vi "ReplaceAllRows_lastrow.vi"(2 "Array in":dbl[][](array[numeric])=[[0.0, 1.0, 2.0], [0.0, 0.0, 0.0], [0.0, 0.0, 0.0], [5.0, 6.0, 7.0]]) -> (0 "Array out":dbl[][](array[numeric])=[[5.0, 6.0, 7.0], [5.0, 6.0, 7.0], [5.0, 6.0, 7.0], [5.0, 6.0, 7.0]])   [LabVIEW 2018]
panel:
  out "last row":dbl[][](array[numeric])=[[5.0, 6.0, 7.0]]
  out "other rows":dbl[][](array[numeric])=[[0.0, 1.0, 2.0], [0.0, 0.0, 0.0], [0.0, 0.0, 0.0]]
  # "the point of this VI is\nto make all rows the same as the last row\nso that anything not modified later is not changed during the ramp"
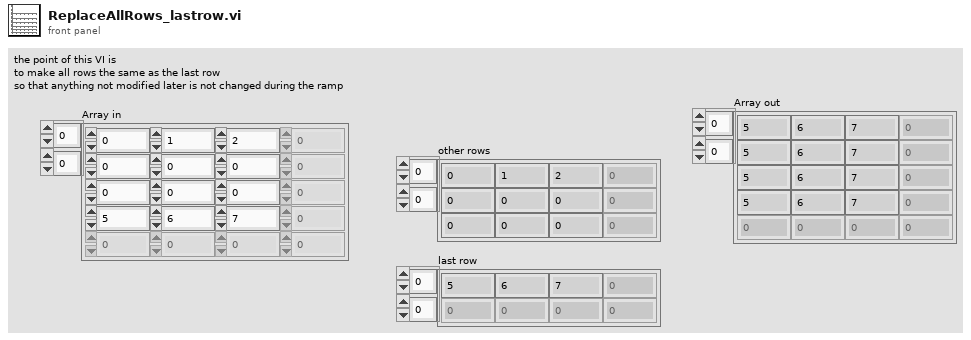
[diagram p1: front panel]
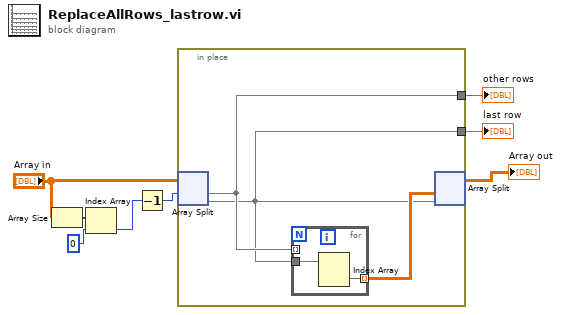
[diagram p0: block diagram]
diagram:
  n1 = Array Size(array="Array in") -> (size(s)=w3:i32[])
  n2 = Index Array(array=w3, index=0) -> (element=w1:i32)
  n3 = Decrement(x=w1) -> (x-1=w5:i32)
  n4 = in-place {
    in-place-border: [w10] -> w7
    in-place-border: [w9] -> w6
    n5 = in-place-split #1("Array in", w5) -> (w10:dbl[][], w9:dbl[][])
    n6 = for {
      tunnel: w10 -> [_] mode=indexing
      tunnel: w9 -> [w13]
      tunnel: [w12] -> w11 mode=indexing
      n7 = Index Array(array=w13) -> (element=w12:dbl[])  [unwired: 2 in]
    }
    n8 = in-place-split #1(w11, w9) -> (→"Array out":dbl[][])  [unwired: 1 out]
  }
  "other rows" <- w7
  "last row" <- w6
